vi "Práctica 6.vi"() -> ()   [LabVIEW 2015]
panel:
  out "Salida":bool
  out "Entrada":bool
  out "Contador":dbl
  out "Estado":T1(ring)
  in  "stop":bool
  out "Cupo lleno":bool
  in  "Fotoselda 2":bool=TRUE
  in  "Fotoselda 1":bool=TRUE
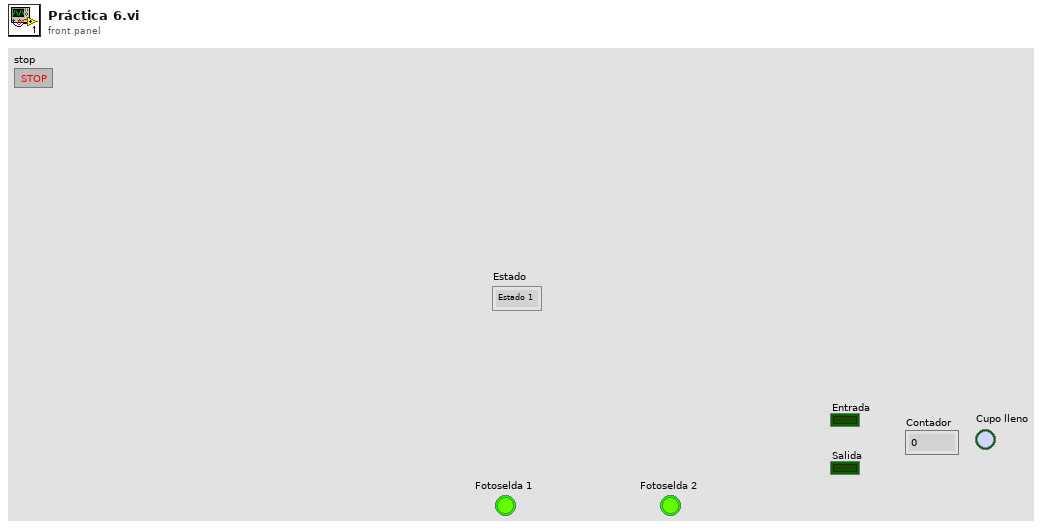
[diagram p1: front panel]
types:
  T1 = enum16{"Estado 1", "Estado 2", "Estado 3", "Estado 4", "Estado 5", "Estado 6", "Estado 7"}
  T2 = enum16{"Estado 1", "Estado 2", "Estado 3", "Estado 4", "Estado 5", "Estado 6", "Esatdo 7"}
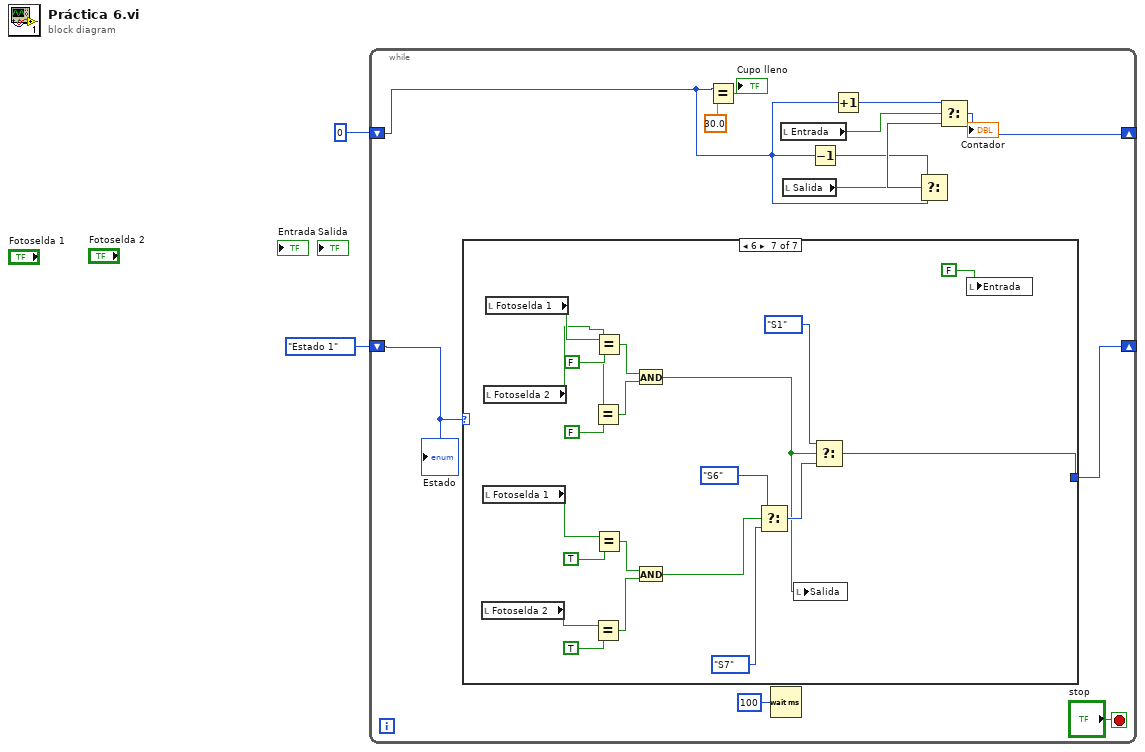
[diagram p0: block diagram]
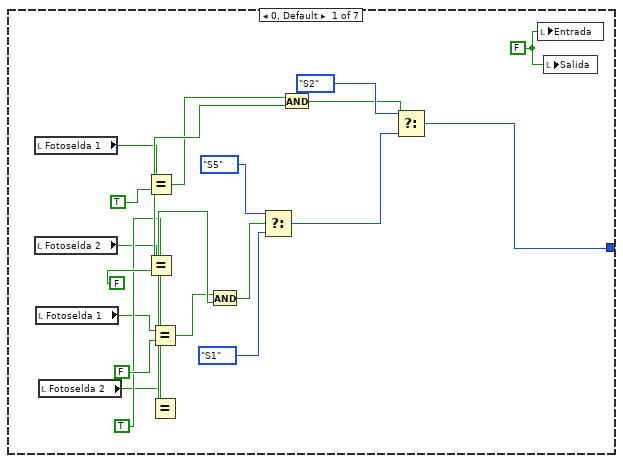
[diagram p2: hidden frame]
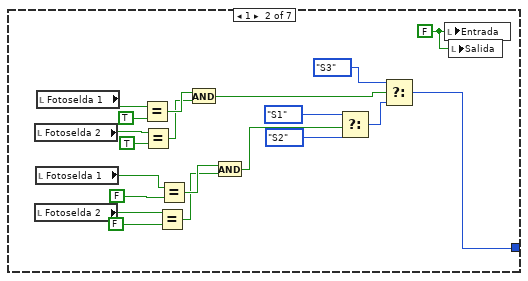
[diagram p3: hidden frame]
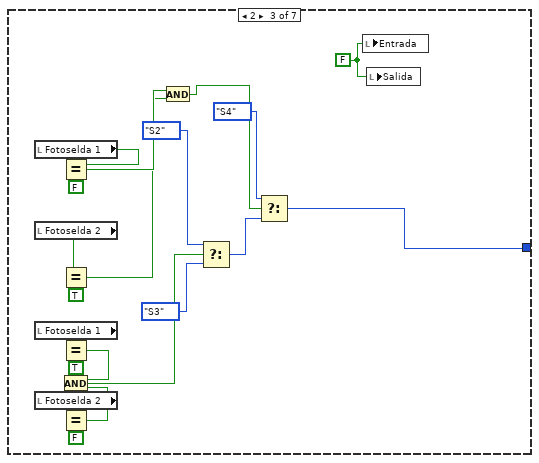
[diagram p4: hidden frame]
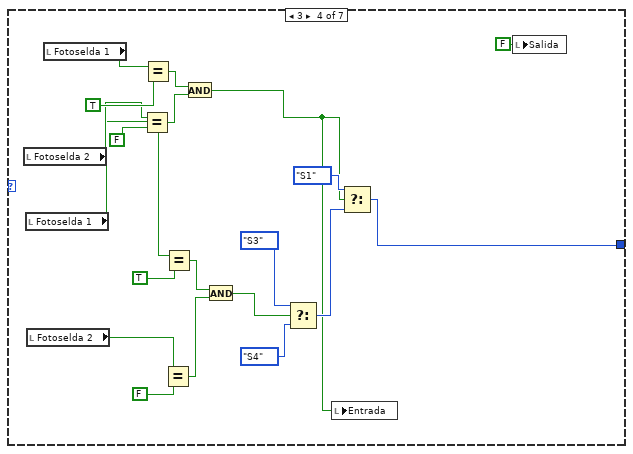
[diagram p5: hidden frame]
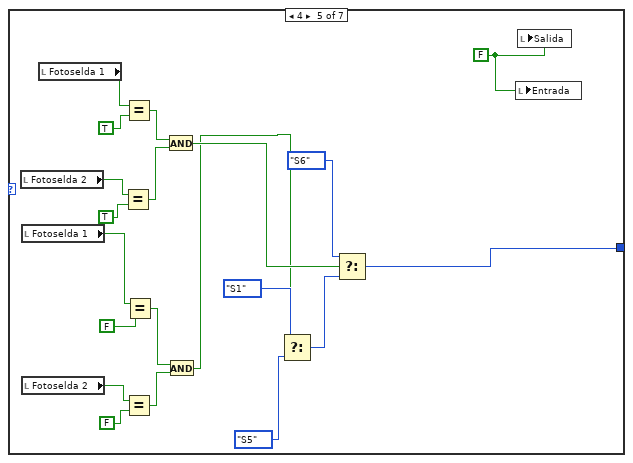
[diagram p6: hidden frame]
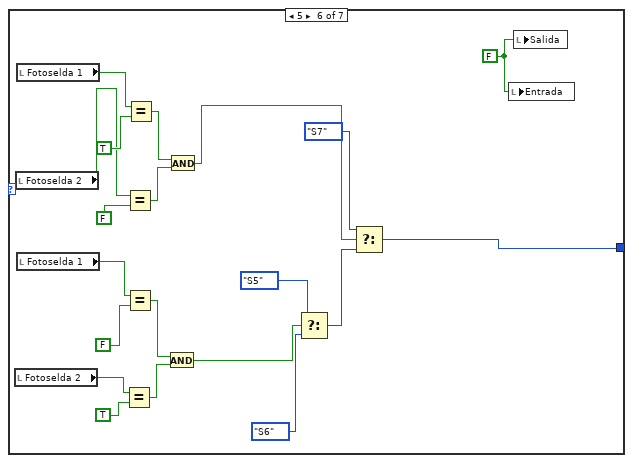
[diagram p7: hidden frame]
diagram:
  n1 = while {
    shift-right: [w13] -> _
    shift-left: T2."Estado 1" ("Enum") -> [w14]
    shift-right: [w8] -> _
    shift-left: 0 -> [w4]
    stop <- "stop" stop-if-true
    n2 = case shown="6" w14 {
      tunnel: [w34 w47 w63 w79 w97 w117 w138] -> w13
      frame 0, Default {
        w16 = FALSE ("x .and. y?")
        n3 = local read "Fotoselda 1"() -> (w21:bool)
        n4 = local read "Fotoselda 2"() -> (w20:bool)
        n5 = local read "Fotoselda 1"() -> (w19:bool)
        n6 = local read "Fotoselda 2"() -> (w18:bool)
        n7 = Equal?(x=w21, y=TRUE) -> (x = y?=w31:bool)
        n8 = Equal?(x=w20, y=FALSE) -> (x = y?=w32:bool)
        n9 = Equal?(x=w19, y=FALSE) -> (x = y?=w26:bool)
        n10 = Equal?(x=w18, y=TRUE) -> (x = y?=w27:bool)
        n11 = And(x=w26, y=w27) -> (x .and. y?=w25:bool)
        n12 = Select(t=enum16{"S1", "S2", "S3", "S4", "S5", "S6", "S7"}."S5" ("Enum"), s=w25, f=enum16{"S1", "S2", "S3", "S4", "S5", "S6", "S7"}."S1" ("Enum")) -> (s? t:f=w29:enum16{"S1", "S2", "S3", "S4", "S5", "S6", "S7"})
        n13 = And(x=w31, y=w32) -> (x .and. y?=w23:bool)
        n14 = Select(t=enum16{"S1", "S2", "S3", "S4", "S5", "S6", "S7"}."S2" ("Enum"), s=w23, f=w29) -> (s? t:f=w34:enum16{"S1", "S2", "S3", "S4", "S5", "S6", "S7"})
        n15 = local write "Entrada"(w16) -> ()
        n16 = local write "Salida"(w16) -> ()
      }
      frame 1 {
        w36 = FALSE ("x .and. y?")
        n17 = local read "Fotoselda 2"() -> (w39:bool)
        n18 = local read "Fotoselda 2"() -> (w41:bool)
        n19 = local read "Fotoselda 1"() -> (w40:bool)
        n20 = local read "Fotoselda 1"() -> (w38:bool)
        n21 = Equal?(x=w38, y=TRUE) -> (x = y?=w46:bool)
        n22 = Equal?(x=w39, y=TRUE) -> (x = y?=w45:bool)
        n23 = Equal?(x=w41, y=FALSE) -> (x = y?=w52:bool)
        n24 = Equal?(x=w40, y=FALSE) -> (x = y?=w53:bool)
        n25 = And(x=w46, y=w45) -> (x .and. y?=w42:bool)
        n26 = And(x=w53, y=w52) -> (x .and. y?=w49:bool)
        n27 = Select(t=enum16{"S1", "S2", "S3", "S4", "S5", "S6", "S7"}."S1" ("Enum"), s=w49, f=enum16{"S1", "S2", "S3", "S4", "S5", "S6", "S7"}."S2" ("Enum")) -> (s? t:f=w54:enum16{"S1", "S2", "S3", "S4", "S5", "S6", "S7"})
        n28 = Select(t=enum16{"S1", "S2", "S3", "S4", "S5", "S6", "S7"}."S3" ("Enum"), s=w42, f=w54) -> (s? t:f=w47:enum16{"S1", "S2", "S3", "S4", "S5", "S6", "S7"})
        n29 = local write "Entrada"(w36) -> ()
        n30 = local write "Salida"(w36) -> ()
      }
      frame 2 {
        w56 = FALSE ("x .and. y?")
        n31 = local read "Fotoselda 1"() -> (w62:bool)
        n32 = local read "Fotoselda 2"() -> (w61:bool)
        n33 = local read "Fotoselda 1"() -> (w60:bool)
        n34 = local read "Fotoselda 2"() -> (w59:bool)
        n35 = Equal?(x=w62, y=FALSE ("Sensor1")) -> (x = y?=w72:bool)
        n36 = Equal?(x=w61, y=TRUE ("Sensor1")) -> (x = y?=w71:bool)
        n37 = Equal?(x=w60, y=TRUE ("Sensor1")) -> (x = y?=w70:bool)
        n38 = Equal?(x=w59, y=FALSE ("Sensor1")) -> (x = y?=w69:bool)
        n39 = And(x=w70, y=w69) -> (x .and. y?=w68:bool)
        n40 = And(x=w72, y=w71) -> (x .and. y?=w58:bool)
        n41 = Select(t=enum16{"S1", "S2", "S3", "S4", "S5", "S6", "S7"}."S2" ("Enum"), s=w68, f=enum16{"S1", "S2", "S3", "S4", "S5", "S6", "S7"}."S3" ("Enum")) -> (s? t:f=w75:enum16{"S1", "S2", "S3", "S4", "S5", "S6", "S7"})
        n42 = Select(t=enum16{"S1", "S2", "S3", "S4", "S5", "S6", "S7"}."S4" ("Enum"), s=w58, f=w75) -> (s? t:f=w63:enum16{"S1", "S2", "S3", "S4", "S5", "S6", "S7"})
        n43 = local write "Entrada"(w56) -> ()
        n44 = local write "Salida"(w56) -> ()
      }
      frame 3 {
        n45 = local read "Fotoselda 2"() -> (w83:bool)
        n46 = local read "Fotoselda 1"() -> (w82:bool)
        n47 = local read "Fotoselda 2"() -> (w81:bool)
        n48 = local read "Fotoselda 1"() -> (w84:bool)
        n49 = Equal?(x=w83, y=FALSE ("Sensor1")) -> (x = y?=w85:bool)
        n50 = Equal?(x=w84, y=TRUE ("Sensor1")) -> (x = y?=w86:bool)
        n51 = Equal?(x=w81, y=FALSE ("Sensor1")) -> (x = y?=w92:bool)
        n52 = Equal?(x=w82, y=TRUE ("Sensor1")) -> (x = y?=w93:bool)
        n53 = And(x=w86, y=w85) -> (x .and. y?=w77:bool)
        n54 = And(x=w93, y=w92) -> (x .and. y?=w91:bool)
        n55 = Select(t=enum16{"S1", "S2", "S3", "S4", "S5", "S6", "S7"}."S3" ("Enum"), s=w91, f=enum16{"S1", "S2", "S3", "S4", "S5", "S6", "S7"}."S4" ("Enum")) -> (s? t:f=w95:enum16{"S1", "S2", "S3", "S4", "S5", "S6", "S7"})
        n56 = local write "Entrada"(w77) -> ()
        n57 = Select(t=enum16{"S1", "S2", "S3", "S4", "S5", "S6", "S7"}."S1" ("Enum"), s=w77, f=w95) -> (s? t:f=w79:enum16{"S1", "S2", "S3", "S4", "S5", "S6", "S7"})
        n58 = local write "Salida"(FALSE ("c--")) -> ()
      }
      frame 4 {
        w96 = FALSE ("c--")
        n59 = local read "Fotoselda 2"() -> (w106:bool)
        n60 = local read "Fotoselda 1"() -> (w100:bool)
        n61 = local read "Fotoselda 2"() -> (w99:bool)
        n62 = local read "Fotoselda 1"() -> (w107:bool)
        n63 = Equal?(x=w106, y=TRUE) -> (x = y?=w110:bool)
        n64 = Equal?(x=w107, y=TRUE) -> (x = y?=w111:bool)
        n65 = Equal?(x=w99, y=FALSE) -> (x = y?=w103:bool)
        n66 = Equal?(x=w100, y=FALSE) -> (x = y?=w104:bool)
        n67 = And(x=w111, y=w110) -> (x .and. y?=w105:bool)
        n68 = And(x=w104, y=w103) -> (x .and. y?=w98:bool)
        n69 = Select(t=enum16{"S1", "S2", "S3", "S4", "S5", "S6", "S7"}."S1" ("Enum"), s=w98, f=enum16{"S1", "S2", "S3", "S4", "S5", "S6", "S7"}."S5" ("Enum")) -> (s? t:f=w115:enum16{"S1", "S2", "S3", "S4", "S5", "S6", "S7"})
        n70 = Select(t=enum16{"S1", "S2", "S3", "S4", "S5", "S6", "S7"}."S6" ("Enum"), s=w105, f=w115) -> (s? t:f=w97:enum16{"S1", "S2", "S3", "S4", "S5", "S6", "S7"})
        n71 = local write "Entrada"(w96) -> ()
        n72 = local write "Salida"(w96) -> ()
      }
      frame 5 {
        w116 = FALSE ("c--")
        n73 = local read "Fotoselda 2"() -> (w118:bool)
        n74 = local read "Fotoselda 2"() -> (w119:bool)
        n75 = local read "Fotoselda 1"() -> (w120:bool)
        n76 = local read "Fotoselda 1"() -> (w121:bool)
        n77 = Equal?(x=w118, y=TRUE) -> (x = y?=w128:bool)
        n78 = Equal?(x=w119, y=FALSE) -> (x = y?=w130:bool)
        n79 = Equal?(x=w121, y=FALSE) -> (x = y?=w129:bool)
        n80 = Equal?(x=w120, y=TRUE) -> (x = y?=w131:bool)
        n81 = And(x=w129, y=w128) -> (x .and. y?=w122:bool)
        n82 = And(x=w131, y=w130) -> (x .and. y?=w123:bool)
        n83 = Select(t=enum16{"S1", "S2", "S3", "S4", "S5", "S6", "S7"}."S5" ("Enum"), s=w122, f=enum16{"S1", "S2", "S3", "S4", "S5", "S6", "S7"}."S6" ("Enum")) -> (s? t:f=w135:enum16{"S1", "S2", "S3", "S4", "S5", "S6", "S7"})
        n84 = Select(t=enum16{"S1", "S2", "S3", "S4", "S5", "S6", "S7"}."S7" ("Enum"), s=w123, f=w135) -> (s? t:f=w117:enum16{"S1", "S2", "S3", "S4", "S5", "S6", "S7"})
        n85 = local write "Entrada"(w116) -> ()
        n86 = local write "Salida"(w116) -> ()
      }
      frame 6 {
        n87 = local read "Fotoselda 2"() -> (w141:bool)
        n88 = local read "Fotoselda 1"() -> (w140:bool)
        n89 = local read "Fotoselda 2"() -> (w142:bool)
        n90 = local read "Fotoselda 1"() -> (w143:bool)
        n91 = Equal?(x=w142, y=FALSE) -> (x = y?=w150:bool)
        n92 = Equal?(x=w141, y=TRUE) -> (x = y?=w148:bool)
        n93 = Equal?(x=w143, y=FALSE) -> (x = y?=w151:bool)
        n94 = Equal?(x=w140, y=TRUE) -> (x = y?=w149:bool)
        n95 = And(x=w151, y=w150) -> (x .and. y?=w137:bool)
        n96 = And(x=w149, y=w148) -> (x .and. y?=w139:bool)
        n97 = Select(t=enum16{"S1", "S2", "S3", "S4", "S5", "S6", "S7"}."S6" ("Enum"), s=w139, f=enum16{"S1", "S2", "S3", "S4", "S5", "S6", "S7"}."S7" ("Enum")) -> (s? t:f=w155:enum16{"S1", "S2", "S3", "S4", "S5", "S6", "S7"})
        n98 = local write "Salida"(w137) -> ()
        n99 = Select(t=enum16{"S1", "S2", "S3", "S4", "S5", "S6", "S7"}."S1" ("Enum"), s=w137, f=w155) -> (s? t:f=w138:enum16{"S1", "S2", "S3", "S4", "S5", "S6", "S7"})
        n100 = local write "Entrada"(FALSE ("c++")) -> ()
      }
    }
    n101 = Equal?(x=w4, y=30.0) -> (x = y?=→"Cupo lleno":bool)
    n102 = Wait (ms)(milliseconds to wait=u32 100) -> ()  [unwired: 1 out]
    n103 = local read "Entrada"() -> (w7:bool)
    n104 = local read "Salida"() -> (w3:bool)
    n105 = Decrement(x=w4) -> (x-1=w5:i32)
    n106 = Increment(x=w4) -> (x+1=w9:i32)
    n107 = Select(t=w5, s=w3, f=w4) -> (s? t:f=w6:i32)
    n108 = Select(t=w9, s=w7, f=w6) -> (s? t:f=w8:i32)
    "Contador" <- w8
    "Estado" <- w14
  }
